vi "SetT0.vi"(8 "error in (no error)":errorcluster, 10 "T0":variant, 11 "PmuBase in":refnum<class "PmuBase.lvclass">) -> (0 "error out":errorcluster, 3 "PmuBase out":refnum<class "PmuBase.lvclass">)   [LabVIEW 2018, in "SensorPlugins.lvlib" / "PmuBase.lvclass"]
uses:
  PmuBase.lvclass
  PmuBase.lvclass/PmuBase.ctl
  Accessors/Read PmuConfig.vi
  Accessors/Write PmuConfig.vi
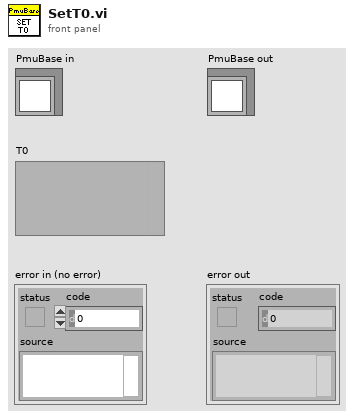
[diagram p1: front panel]
types:
  T1 = typedef "SensorPlugins.lvlib/PmuBase.lvclass/PmuConfig.ctl" = cluster{"Class":enum16{"M", "P"}, "Fs":i32, "F0":i32, "FSamp":i32, "SettlingTime":dbl, "T0":ext}
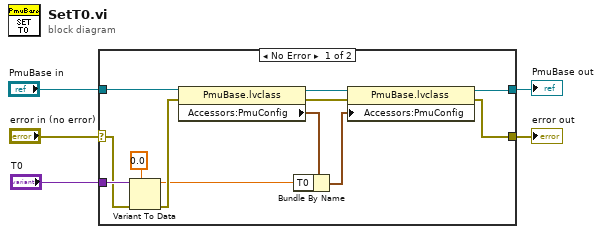
[diagram p0: block diagram]
diagram:
  n1 = case shown="No Error" "error in (no error)" {
    selector: "error in (no error)" -> [w14 w18]
    tunnel: "PmuBase in" -> [w17 w19]
    tunnel: [w7 w19] -> w3
    tunnel: [w6 w18] -> w2
    tunnel: "T0" -> [w16 _]
    frame No Error {
      n2 = Variant To Data(error in=w14, type=0.0, Variant=w16) -> (data=w11:dbl, error out=w13:errorcluster)
      n3 = property class="PmuBase.lvclass"(reference=w17, error in=w13) -> (reference out=w10:refnum<class "PmuBase.lvclass">, error out=w8:errorcluster, "Accessors:PmuConfig"=w12:T1)
      n4 = Bundle By Name(cluster=w12, "T0"=w11) -> (w9:T1)
      n5 = property class="PmuBase.lvclass"(reference=w10, error in=w8, "Accessors:PmuConfig"=w9) -> (reference out=w7:refnum<class "PmuBase.lvclass">, error out=w6:errorcluster)
    }
    frame Error {
    }
  }
  "error out" <- w2
  "PmuBase out" <- w3
